vi "Nested Name.vi"() -> (2 "Nested Name":string)   [LabVIEW 2021, in "Ex Queue Actor.lvlib" / "Ex Queue Actor.lvclass"]
uses:
  Ex Queue Actor.lvclass
  Ex Queue Actor.lvclass/Ex Queue Actor.ctl
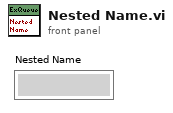
[diagram p1: front panel]
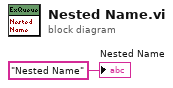
[diagram p0: block diagram]
diagram:
  "Nested Name" <- "Nested Name" ("Nested Name")
